vi "Write_Growth_DB.vi"(0 "Growth Name":string, 1 "Notes":string, 2 "Log File":path, 3 "Growth Sequence File":path, 4 "Operator Name":string) -> (5 "Error":bool)   [LabVIEW 2011]
uses:
  low_level_proc/globals.vi
panel:
  out "concatenated string":string
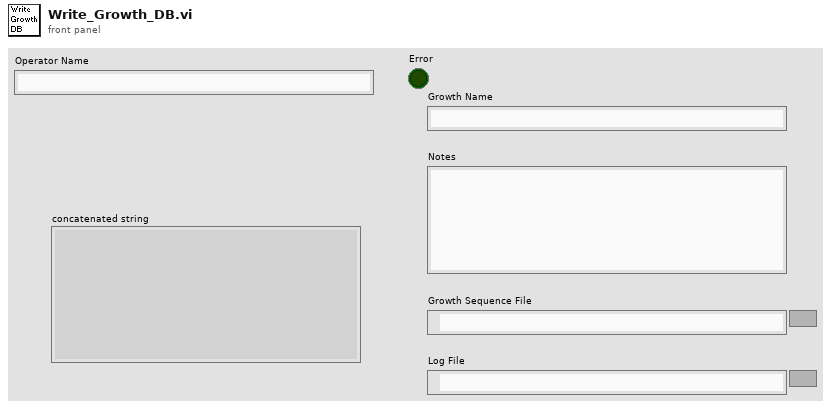
[diagram p1: front panel]
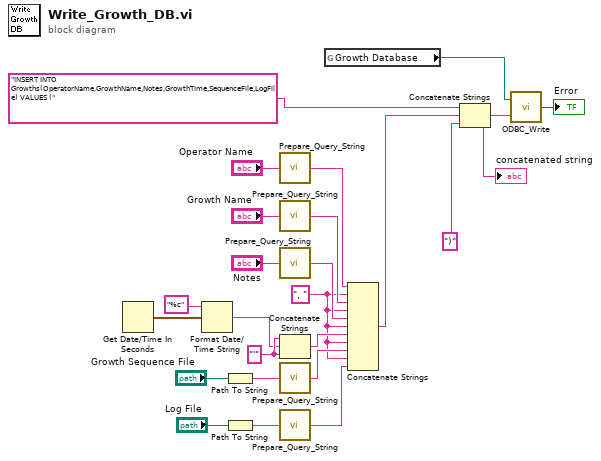
[diagram p0: block diagram]
diagram:
  w6 = "'" ("string")
  w2 = ", " ("string")
  n1 = Get Date/Time In Seconds() -> (seconds since 1Jan1904=w8:timestamp)
  n2 = Format Date/Time String(time format string (%c)="%c", seconds (now)=w8) -> (date/time string=w5:string)  [unwired: 1 in]
  n3 = Path To String(path="Growth Sequence File") -> (string=w16:string)
  n4 = Path To String(path="Log File") -> (string=w14:string)
  n5 = call "Prepare_Query_String.vi"("Input String"="Operator Name") -> ("Output String"=w12:string)
  n6 = call "Prepare_Query_String.vi"("Input String"="Growth Name") -> ("Output String"=w11:string)
  n7 = call "Prepare_Query_String.vi"("Input String"="Notes") -> ("Output String"=w9:string)
  n8 = Concatenate Strings(w6, w5, w6) -> (w4:string)
  n9 = call "Prepare_Query_String.vi"("Input String"=w16) -> ("Output String"=w3:string)
  n10 = call "Prepare_Query_String.vi"("Input String"=w14) -> ("Output String"=w1:string)
  n11 = global read "globals.vi" "Growth Database"() -> (w20:path)
  n12 = Concatenate Strings(w12, w2, w11, w2, w9, w2, w4, w2, w3, w2, w1) -> (w10:string)
  n13 = Concatenate Strings("INSERT INTO Growths(OperatorName,GrowthName,Notes,GrowthTime,SequenceFile,LogFile) VALUES (" ("string"), w10, ")" ("string")) -> (w23:string)
  "concatenated string" <- w23
  n14 = call "ODBC_Write.vi"("Query"=w23, "Database File"=w20) -> ("Error"=→"Error":bool)
